vi "Example Collection Client-Server.vi"() -> ()   [LabVIEW 2013]
uses:
  Connection/Connection.lvclass
  Connection.TCP/Connection.TCP.lvclass
  Connection.Collection/Connection.Collection.lvclass
  Connection.LocalQueue/Connection.LocalQueue.lvclass
panel:
  out "Values":dbl[](array[numeric])
  out "Echo matches":bool[](array[boolean])
  out "Errors 3":errorcluster[](array[cluster])
  out "Numeric":i32
  in  "stop":bool
  out "connected":bool
  out "Classes":string[](array[string])
  out "listener error":errorcluster
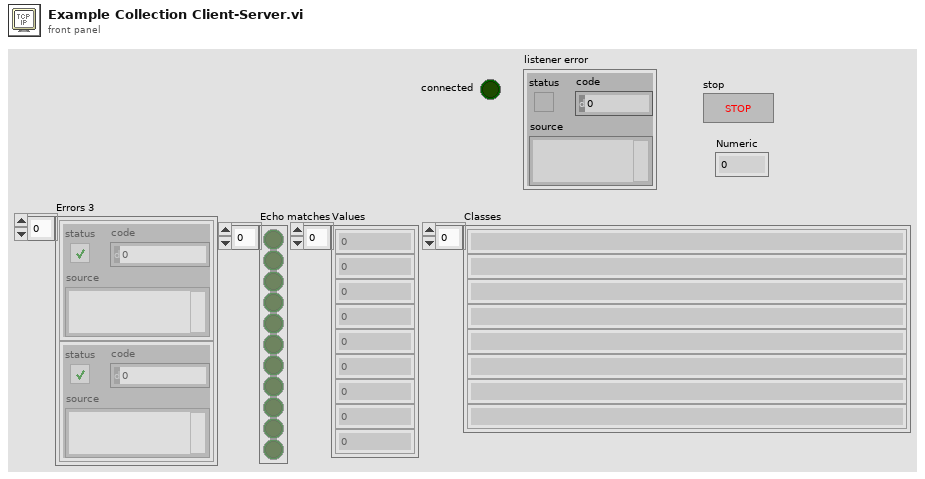
[diagram p1: front panel]
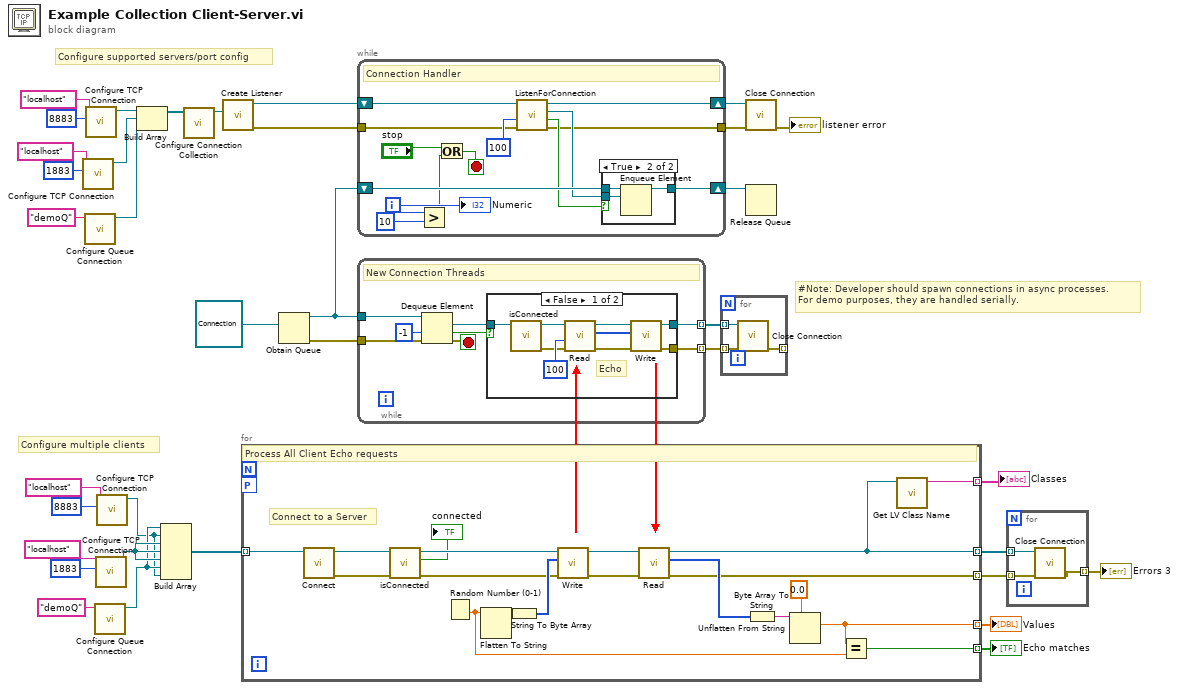
[diagram p0: block diagram]
diagram:
  # "#Note: Developer should spawn connections in async processes.\nFor demo purposes, they are handled serially."
  # "Configure multiple clients"
  # "Configure supported servers/port config"
  n1 = call "Configure TCP Connection.vi"("remote port (80)"=u16 1883, "address (localhost)"="localhost") -> ("Connection.TCP"=w27:refnum<class "Connection.TCP.lvclass">)  [unwired: 8 in, 1 out]
  n2 = call "Configure Queue Connection.vi"("Queue Name"="demoQ") -> ("Connection.LocalQueue"=w11:refnum<class "Connection.LocalQueue.lvclass">)  [unwired: 9 in, 1 out]
  n3 = call "Configure TCP Connection.vi"("remote port (80)"=u16 8883, "address (localhost)"="localhost") -> ("Connection.TCP"=w31:refnum<class "Connection.TCP.lvclass">)  [unwired: 8 in, 1 out]
  n4 = call "Configure Queue Connection.vi"("Queue Name"="demoQ") -> ("Connection.LocalQueue"=w8:refnum<class "Connection.LocalQueue.lvclass">)  [unwired: 9 in, 1 out]
  n5 = call "Configure TCP Connection.vi"("remote port (80)"=u16 1883, "address (localhost)"="localhost") -> ("Connection.TCP"=w9:refnum<class "Connection.TCP.lvclass">)  [unwired: 8 in, 1 out]
  n6 = call "Configure TCP Connection.vi"("remote port (80)"=u16 8883, "address (localhost)"="localhost") -> ("Connection.TCP"=w7:refnum<class "Connection.TCP.lvclass">)  [unwired: 8 in, 1 out]
  n7 = Build Array(w31, w27, w11) -> (w32:refnum<class "Connection.lvclass">[])
  n8 = Build Array(w8, w7, w9, w9, w9, w8, w7) -> (w5:refnum<class "Connection.lvclass">[])
  n9 = call "Configure Connection Collection.vi"("Collection"=w32) -> ("Connection"=w30:refnum<class "Connection.Collection.lvclass">)  [unwired: 9 in, 1 out]
  n10 = call "Create Listener.vi"("Connection Configuration"=w30) -> ("error out"=w20:errorcluster, "Listener"=w21:refnum<class "Connection.lvclass">)  [unwired: 9 in]
  n11 = for {
    tunnel: [w38] -> w24 mode=indexing
    tunnel: [w43] -> w13 mode=indexing
    tunnel: w5 -> [w41] mode=indexing
    tunnel: [w40] -> w4 mode=indexing
    tunnel: [w39] -> w3 mode=indexing
    workers-P: _ -> [_]
    tunnel: [w37] -> w1 mode=indexing
    # "Connect to a Server"
    # "Process All Client Echo requests"
    n12 = call "Connect.vi"("Connection in"=w41) -> ("error out"=w48:errorcluster, "Connection out"=w46:refnum<class "Connection.lvclass">)  [unwired: 9 in]
    n13 = call "isConnected.vi"("error in (no error)"=w48, "Connection in"=w46) -> ("error out"=w47:errorcluster, "connected"=→"connected":bool, "Connection out"=w45:refnum<class "Connection.lvclass">)  [unwired: 7 in]
    n14 = Random Number (0-1)() -> (number: 0 to 1=w49:dbl)
    n15 = Flatten To String(anything=w49) -> (data string=w54:string)  [unwired: 3 in, 2 out]
    n16 = String To Byte Array(string=w54) -> (unsigned byte array=w53:u8[])
    n17 = call "Write.vi"("error in (no error)"=w47, "Bytes"=w53, "Connection in"=w45) -> ("error out"=w44:errorcluster, "Connection"=w55:refnum<class "Connection.lvclass">)  [unwired: 7 in]
    n18 = call "Read.vi"("error in (no error)"=w44, "TCPConnection in"=w55) -> ("error out"=w43:errorcluster, "Bytes"=w52:u8[], "TCPConnection out"=w38:refnum<class "Connection.lvclass">)  [unwired: 5 in, 2 out]
    n19 = Byte Array To String(unsigned byte array=w52) -> (string=w51:string)
    n20 = Unflatten From String(type=0.0, binary string=w51) -> (value=w39:dbl)  [unwired: 3 in, 2 out]
    n21 = Equal?(x=w39, y=w49) -> (x = y?=w40:bool)
    n22 = call <vilib>:"Get LV Class Name.vi"("object"=w38) -> ("class name"=w37:string)  [unwired: 9 in, 1 out]
  }
  "Classes" <- w1
  "Echo matches" <- w4
  "Values" <- w3
  n23 = Obtain Queue(element data type=refnum<class "Connection.lvclass"> refnum ("Connection")) -> (queue out=w16:refnum<queue>, error out=w15:errorcluster)  [unwired: 4 in, 1 out]
  n24 = while {
    shift-right: [w66] -> w22
    shift-left: w16 -> [w67]
    tunnel: w20 -> [w63]
    tunnel: [w61] -> w18
    shift-right: [w62] -> w19
    shift-left: w21 -> [w68]
    i -> [w58]
    stop <- w60 stop-if-true
    # "Connection Handler"
    n25 = Greater?(x=w58, y=10) -> (0:w56:bool)
    n26 = Or(x="stop", y=w56) -> (x .or. y?=w60:bool)
    n27 = call "ListenForConnection.vi"("error in (no error)"=w63, "timeout (2000 ms)"=100 ("bytes to read (100)"), "Listener"=w68) -> ("error out"=w61:errorcluster, "New connection"=w64:bool, "Connection"=w65:refnum<class "Connection.lvclass">, "Listener out"=w62:refnum<class "Connection.lvclass">)  [unwired: 5 in]
    n28 = case shown="True" w64 {
      tunnel: w67 -> [w70 w73]
      tunnel: [w70 w72] -> w66
      tunnel: w65 -> [_ w71]
      frame False {
      }
      frame True {
        n29 = Enqueue Element(queue=w73, element=w71) -> (queue out=w72:refnum<queue>)  [unwired: 2 in, 2 out]
      }
    }
    "Numeric" <- w58
  }
  n30 = while {
    tunnel: [w81] -> w2 mode=indexing
    tunnel: w16 -> [w80]
    tunnel: w15 -> [w78]
    tunnel: [w74] -> w14 mode=indexing
    stop <- w75 stop-if-true
    # "New Connection Threads"
    n31 = Dequeue Element(queue=w80, timeout in ms (-1)=-1, error in (no error)=w78) -> (element=w77:refnum<class "Connection.lvclass">, timed out?=w76:bool, error out=w75:errorcluster)  [unwired: 1 out]
    n32 = case shown="False" w76 {
      tunnel: [w84 _] -> w81
      tunnel: w77 -> [w86 _]
      tunnel: [w82 _] -> w74
      frame False {
        # "Echo"
        n33 = call "isConnected.vi"("Connection in"=w86) -> ("error out"=w87:errorcluster, "Connection out"=w88:refnum<class "Connection.lvclass">)  [unwired: 8 in, 1 out]
        n34 = call "Read.vi"("error in (no error)"=w87, "timeout (2000 ms)"=100 ("bytes to read (100)"), "TCPConnection in"=w88) -> ("error out"=w83:errorcluster, "Bytes"=w85:u8[], "TCPConnection out"=w89:refnum<class "Connection.lvclass">)  [unwired: 4 in, 2 out]
        n35 = call "Write.vi"("error in (no error)"=w83, "Bytes"=w85, "Connection in"=w89) -> ("error out"=w84:errorcluster, "Connection"=w82:refnum<class "Connection.lvclass">)  [unwired: 7 in]
      }
      frame True {
      }
    }
  }
  n36 = for {
    tunnel: w14 -> [w93] mode=indexing
    tunnel: [w92] -> _ mode=indexing
    tunnel: w2 -> [w91] mode=indexing
    n37 = call "Close Connection.vi"("error in (no error)"=w91, "Connection in"=w93) -> ("error out"=w92:errorcluster)  [unwired: 8 in, 1 out]
  }
  n38 = call "Close Connection.vi"("error in (no error)"=w18, "Connection in"=w19) -> ("error out"=→"listener error":errorcluster)  [unwired: 8 in, 1 out]
  n39 = Release Queue(queue=w22) -> ()  [unwired: 2 in, 3 out]
  n40 = for {
    tunnel: w24 -> [w96] mode=indexing
    tunnel: w13 -> [w95] mode=indexing
    tunnel: [w94] -> w6 mode=indexing
    n41 = call "Close Connection.vi"("error in (no error)"=w95, "Connection in"=w96) -> ("error out"=w94:errorcluster)  [unwired: 8 in, 1 out]
  }
  "Errors 3" <- w6
